vi "ValidateVariableArrayJSON.vi"(8 "error in (no error)":errorcluster, 11 "JSONVariableArray":string) -> (0 "error out":errorcluster, 1 "Valid Count":i32, 2 "InvalidVariables?":bool, 3 "JSONVarSet":T1, 4 "JSONErrorResponse":string)   [LabVIEW 2013]
doc: "Checks the contents of a JSON array for objects corresponding to valid SetList variable representations. Generates error messages and discards those that do not.\n\nThis enables checking basic structure and giving appropriate results to the client without having to actually apply the variables."
uses:
  JSONVarSet.ctl
  <vilib>/regexp/Match Regular Expression.xnode
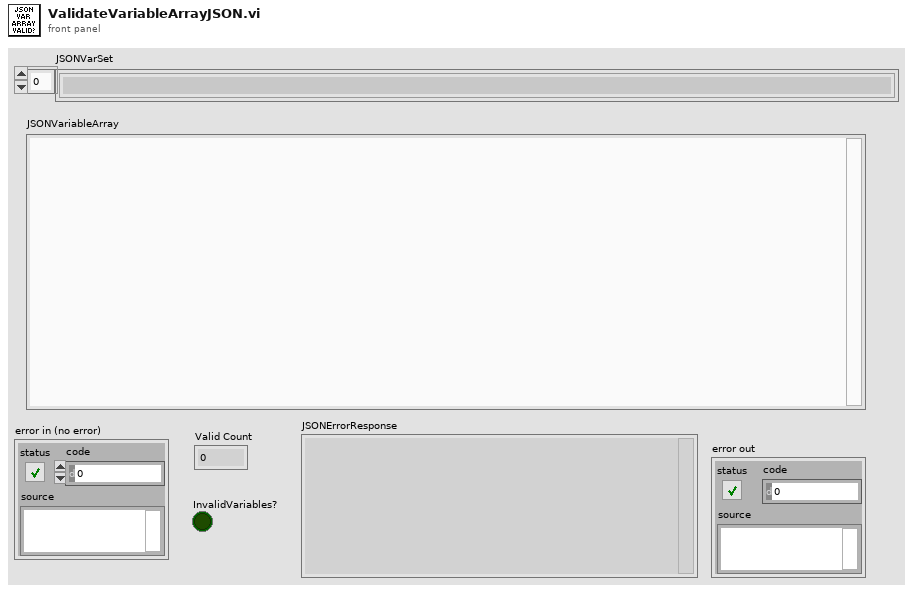
[diagram p1: front panel]
types:
  T1 = typedef "JSONVarSet.ctl" = string[]
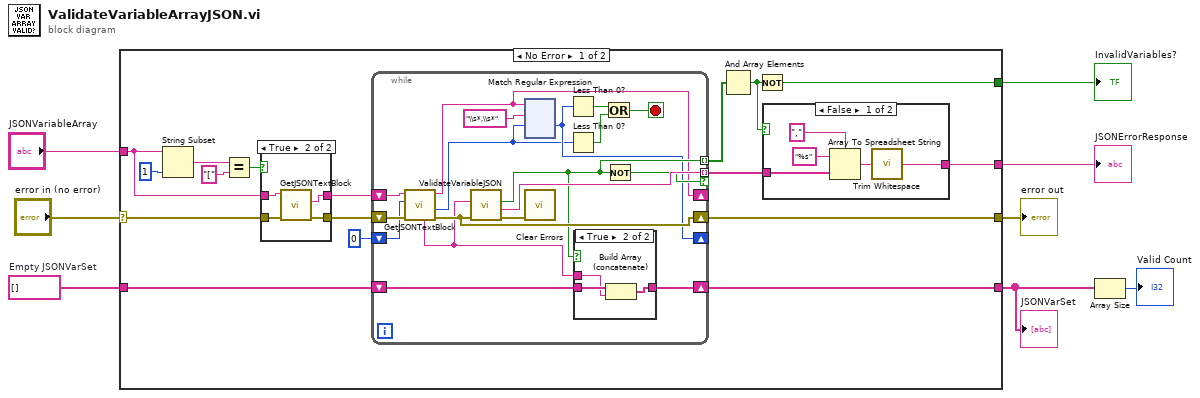
[diagram p0: block diagram]
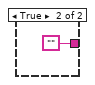
[diagram p2: hidden frame]
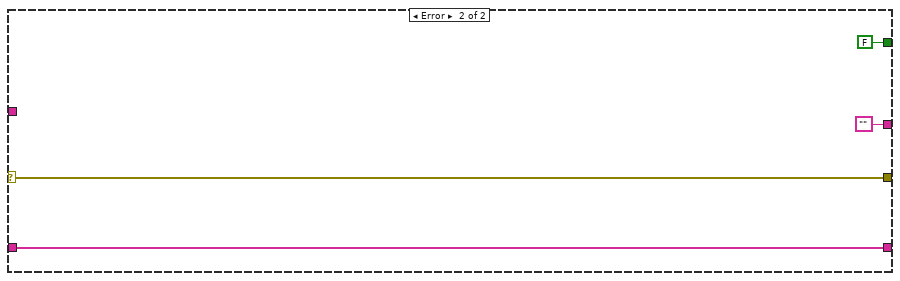
[diagram p5: hidden frame]
diagram:
  w6 = T1 []  # Empty JSONVarSet
  n1 = case shown="No Error" "error in (no error)" {
    selector: "error in (no error)" -> [w18 w177]
    tunnel: "JSONVariableArray" -> [w23 _]
    tunnel: [w25 w176] -> w5
    tunnel: [w24 w177] -> w7
    tunnel: w6 -> [w15 w176]
    tunnel: [w12 ""] -> w3
    tunnel: [w10 FALSE] -> w2
    frame No Error {
      n2 = String Subset(string=w23, length (rest)=1 ("length (rest)")) -> (substring=w21:string)  [unwired: 1 in]
      n3 = Equal?(x=w21, y="[") -> (x = y?=w19:bool)
      n4 = case shown="True" w19 {
        tunnel: [w33 w37] -> w9
        tunnel: w23 -> [w33 w36]
        tunnel: w18 -> [w32 w35]
        tunnel: [w32 w34] -> w17
        frame False {
        }
        frame True {
          n5 = call "GetJSONTextBlock.vi"("error in (no error)"=w35, "String In"=w36) -> ("error out"=w34:errorcluster, "Matched Block Contents"=w37:string)  [unwired: 5 in, 3 out]
        }
      }
      n6 = while {
        shift-right: [w42] -> _
        shift-left: w9 -> [w53]
        shift-right: [w43] -> _
        shift-left: 0 ("offset past token") -> [w54]
        shift-right: [w49] -> w25
        shift-left: w15 -> [w48]
        shift-right: [w51] -> w24
        shift-left: w17 -> [w55]
        tunnel: [w45] -> w14 mode=indexing
        tunnel: [w52] -> w13 mode=indexing if=w46
        stop <- w38 stop-if-true
        n7 = call "GetJSONTextBlock.vi"("error in (no error)"=w55, "Block Start Offset"=w54, "String In"=w53) -> ("error out"=w51:errorcluster, "Offset Past Block"=w41:i32, "String Out"=w42:string, "Matched Block"=w47:string)  [unwired: 4 in, 1 out]
        n8 = call "ValidateVariableJSON.vi"("error in (no error)"=w51, "JSON Variable Object"=w47) -> ("error out"=w50:errorcluster, "JSON Error String"=w52:string, "Valid?"=w45:bool)  [unwired: 7 in]
        n9 = xnode "Match Regular Expression"("input string"=w42, "regular expression"="\\s*,\\s*", "offset (0)"=w41) -> ("offset past match"=w43:i32)  [unwired: 3 in, 4 out]
        n10 = call <vilib>:"Clear Errors.vi"("error in (no error)"=w50) -> ()  [unwired: 6 in, 1 out]
        n11 = Less Than 0?(x=w43) -> (x < 0?=w40:bool)
        n12 = Less Than 0?(x=w41) -> (x < 0?=w39:bool)
        n13 = case shown="True" w45 {
          tunnel: [w170 w173] -> w49
          tunnel: w48 -> [w170 w172]
          tunnel: w47 -> [_ w171]
          frame False {
          }
          frame True {
            n14 = Build Array (concatenate)(w172, w171) -> (w173:T1)
          }
        }
        n15 = Or(x=w40, y=w39) -> (x .or. y?=w38:bool)
        n16 = Not(x=w45) -> (.not. x?=w46:bool)
      }
      n17 = And Array Elements(Boolean array=w14) -> (logical AND=w11:bool)
      n18 = Not(x=w11) -> (.not. x?=w10:bool)
      n19 = case shown="False" w11 {
        tunnel: w13 -> [w28 _]
        tunnel: [w26 ""] -> w12
        frame False {
          n20 = Array To Spreadsheet String(delimiter (Tab)=",", array=w28, 3:"%s" ("format string")) -> (spreadsheet string=w27:string)
          n21 = call <vilib>:"Trim Whitespace.vi"("string"=w27) -> ("trimmed string"=w26:string)  [unwired: 1 in]
        }
        frame True {
        }
      }
    }
    frame Error {
    }
  }
  "JSONVarSet" <- w5
  "error out" <- w7
  "JSONErrorResponse" <- w3
  "InvalidVariables?" <- w2
  n22 = Array Size(array=w5) -> (size(s)=→"Valid Count":i32)
